vi "VIE.Module.Queued Message Handler.dqClass_dataProbe.vi"(1 "data":T1) -> (0 "Boolean":bool)   [LabVIEW 2010, in "VIE.Module.Queued Message Handler.QueuedMessageHandler.dqGOOPClass.lvlib"]
doc: "Use this custom probe to probe a dqGOOP object data cluster. Conditions can be created that are useful for your particular class. Be sure to move or copy this VI to the user.lib\\_probes or the Default Data\\Probes directories."
uses:
  VIE.Module.Queued Message Handler.QueuedMessageHandler.dqGOOPClass.lvlib
  VIE.Module.Queued Message Handler.dqClass_ObjectData.ctl
panel:
  in  "Tab Control":enum32{"data", "condition"}(tab)
  out "data":T1
  # "Pause if any of the following:"
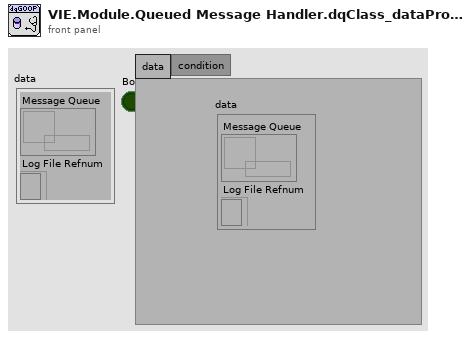
[diagram p1: front panel]
types:
  T1 = typedef "VIE.Module.Queued Message Handler.QueuedMessageHandler.dqGOOPClass.lvlib/VIE.Module.Queued Message Handler.dqClass_ObjectData.ctl" = cluster{"Message Queue":refnum<queue>, "Log File Refnum":refnum<file>}
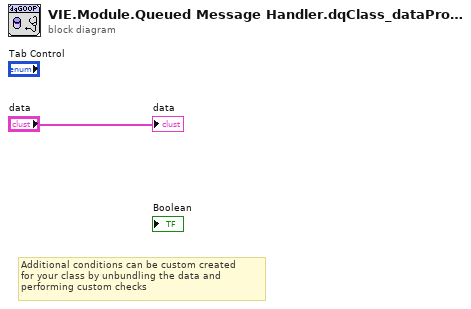
[diagram p0: block diagram]
diagram:
  # "Additional conditions can be custom created\nfor your class by unbundling the data and\nperforming custom checks"
  "data" <- "data"
